vi "DeviceNet Display.vi"() -> ()   [LabVIEW 2011]
uses:
  Controls/DNet CommandRegister Cluster.ctl
  GlobalVariables.vi
panel:
  in  "Enable Write":bool
  out "DNET3":string
  out "DNET2":string
  out "DNET1":string
  in  "stop":bool
  in  "Reset":bool
  in  "HaltScanner":bool
  in  "DisableNetwork":bool
  in  "Fault":bool
  out "DnetPowerDetect":bool
  out "DupNodeFail":bool
  out "CommFailure":bool
  out "Autoverify":bool
  out "DeviceFailure":bool
  out "DisableNetwork":bool
  out "Fault":bool
  out "Run":bool
  in  "Run":bool
  in  "Reset":bool
  in  "HaltScanner":bool
  in  "DisableNetwork":bool
  in  "Fault":bool
  out "DnetPowerDetect":bool
  out "DupNodeFail":bool
  out "CommFailure":bool
  out "Autoverify":bool
  out "DeviceFailure":bool
  out "DisableNetwork":bool
  out "Fault":bool
  out "Run":bool
  in  "Run":bool
  in  "Reset":bool
  in  "HaltScanner":bool
  in  "DisableNetwork":bool
  in  "Fault":bool
  out "DnetPowerDetect":bool
  out "DupNodeFail":bool
  out "CommFailure":bool
  out "Autoverify":bool
  out "DeviceFailure":bool
  out "DisableNetwork":bool
  out "Fault":bool
  out "Run":bool
  in  "Run":bool
  # "DeviceNet 1"
  # "DeviceNet 2"
  # "DeviceNet 3"
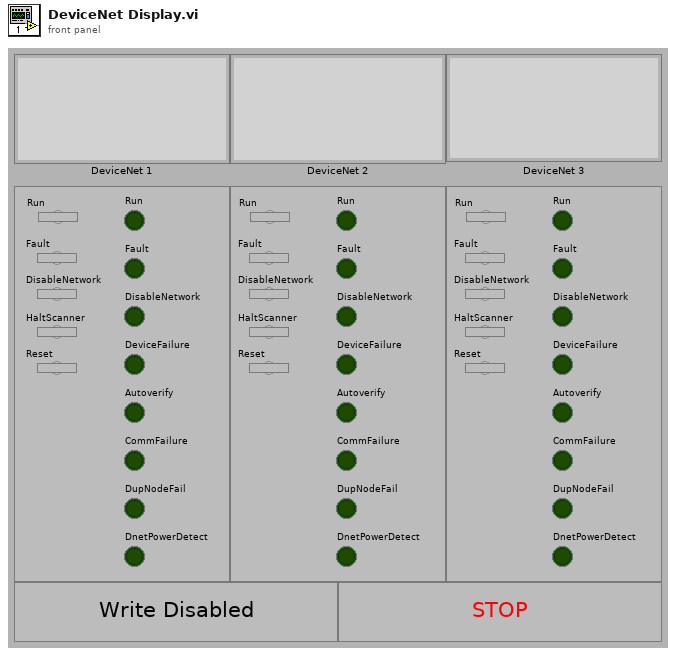
[diagram p1: front panel]
types:
  T1 = typedef "DNet CommandRegister Cluster.ctl" = cluster{"Run":bool, "Fault":bool, "DisableNetowrk":bool, "HaltScanner":bool, "Reset":bool}
  T2 = typedef "DNet StatusRegister Cluster.ctl" = cluster{"Run":bool, "Fault":bool, "DisableNetwork":bool, "DeviceFailure":bool, "Autoverify":bool, "CommFailure":bool, "DupNodeFail":bool, "DnetPowerDetect":bool}
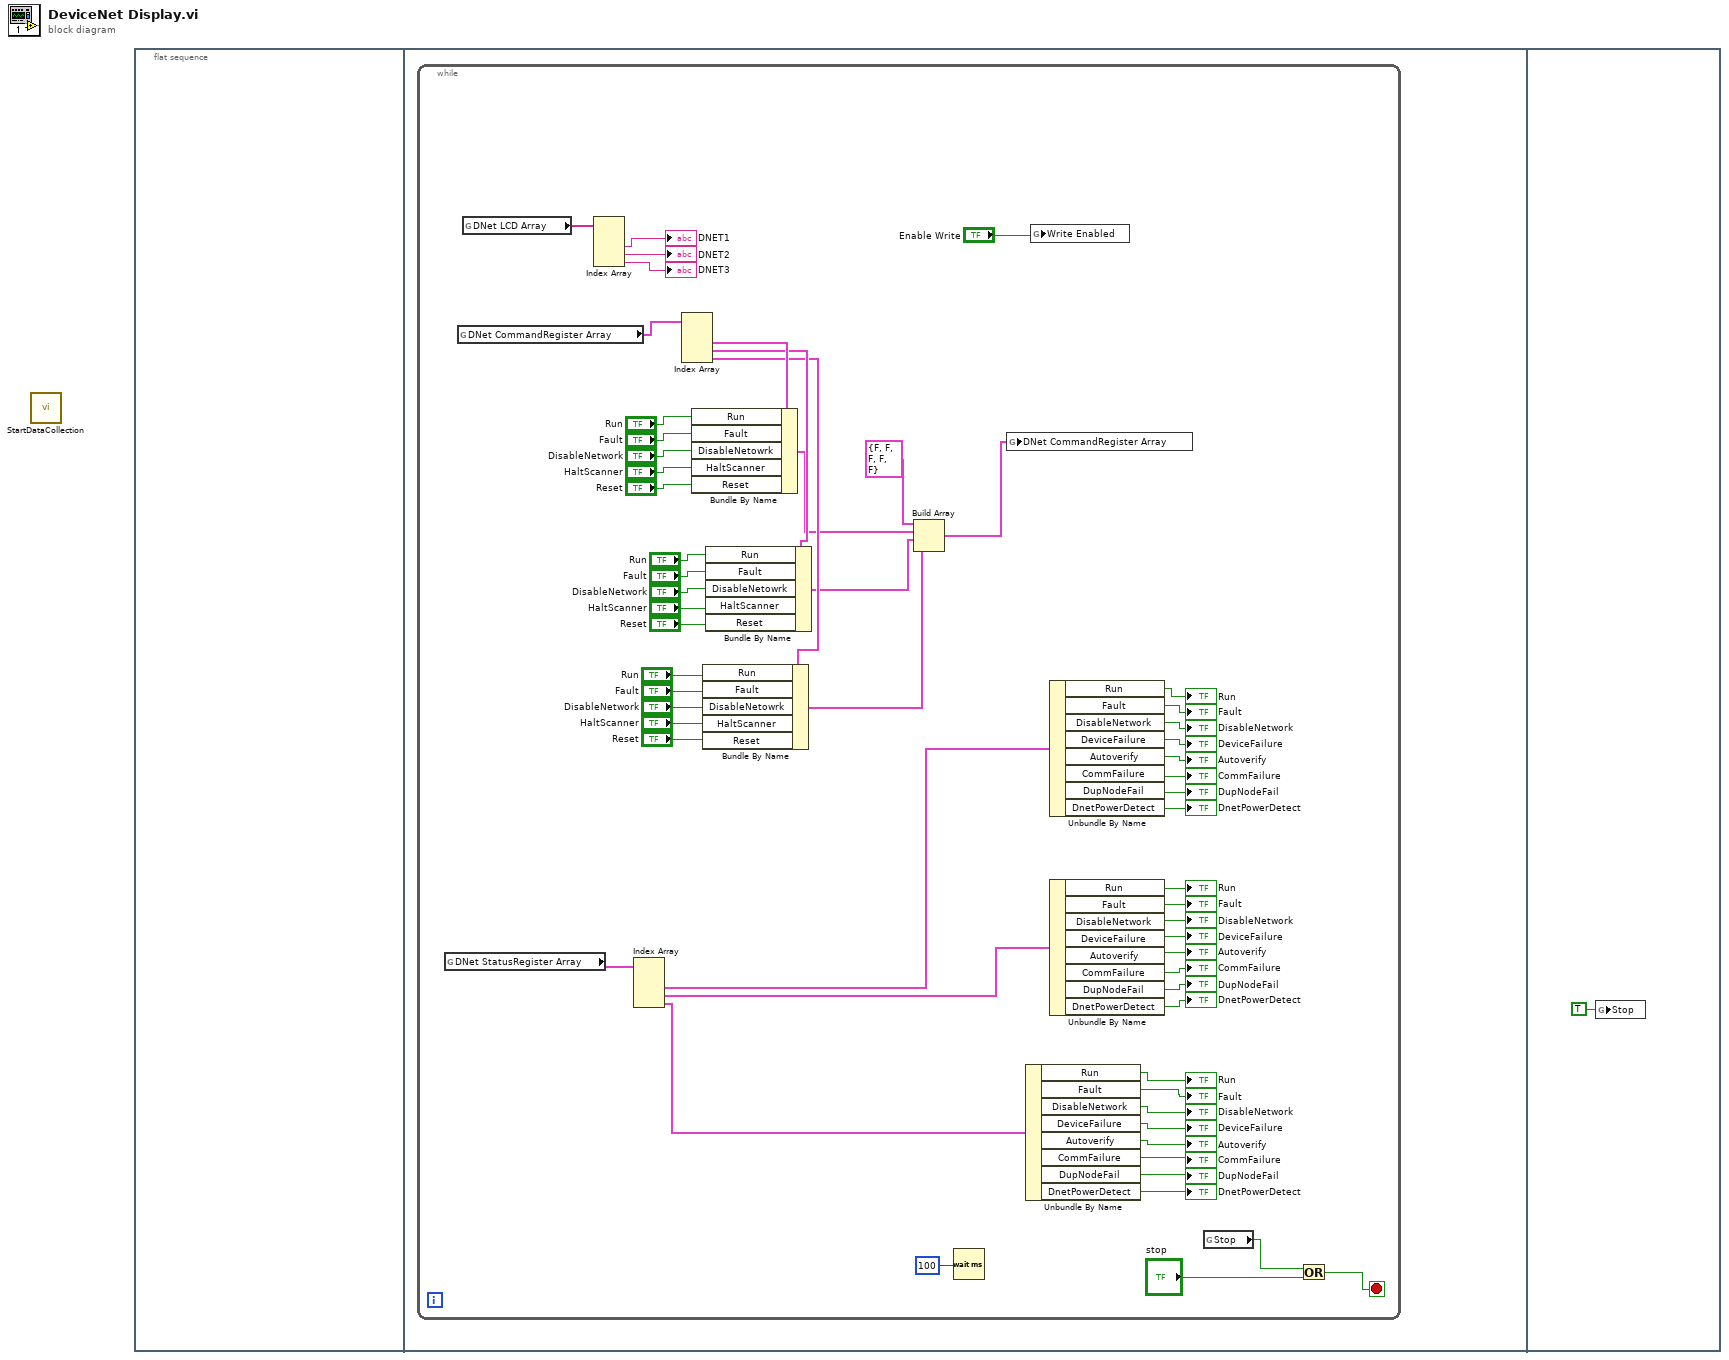
[diagram p0: block diagram]
diagram:
  n1 = call "StartDataCollection.vi"() -> ()  [unwired: 12 in]
  n2 = flat-sequence {
    frame #0 {
    }
    frame #1 {
      n3 = while {
        stop <- w2 stop-if-true
        n4 = global read "GlobalVariables.vi" "DNet StatusRegister Array"() -> (w33:T2[])
        n5 = global read "GlobalVariables.vi" "DNet CommandRegister Array"() -> (w55:T1[])
        n6 = global read "GlobalVariables.vi" "DNet LCD Array"() -> (w60:string[])
        n7 = Index Array(array=w60) -> (element #2=→"DNET1":string, element #3=→"DNET2":string, element #4=→"DNET3":string)  [unwired: 4 in, 1 out]
        n8 = Index Array(array=w33) -> (element #2=w32:T2, element #3=w31:T2, element #4=w30:T2)  [unwired: 4 in, 1 out]
        n9 = Index Array(array=w55) -> (element #2=w56:T1, element #3=w54:T1, element #4=w53:T1)  [unwired: 4 in, 1 out]
        n10 = Bundle By Name(cluster=w56, "Run"="Run", "Fault"="Fault", "DisableNetowrk"="DisableNetwork", "HaltScanner"="HaltScanner", "Reset"="Reset") -> (w37:T1)
        n11 = Bundle By Name(cluster=w53, "Run"="Run", "Fault"="Fault", "DisableNetowrk"="DisableNetwork", "HaltScanner"="HaltScanner", "Reset"="Reset") -> (w35:T1)
        n12 = Bundle By Name(cluster=w54, "Run"="Run", "Fault"="Fault", "DisableNetowrk"="DisableNetwork", "HaltScanner"="HaltScanner", "Reset"="Reset") -> (w36:T1)
        n13 = Build Array(T1 {"Run"=FALSE, "Fault"=FALSE, "DisableNetowrk"=FALSE, "HaltScanner"=FALSE, "Reset"=FALSE} ("element"), w37, w36, w35) -> (w34:T1[])
        n14 = Wait (ms)(milliseconds to wait=100) -> ()  [unwired: 1 out]
        n15 = global write "GlobalVariables.vi" "DNet CommandRegister Array"(w34) -> ()
        n16 = Unbundle By Name(w30) -> ("Run"=→"Run":bool, "Fault"=→"Fault":bool, "DisableNetwork"=→"DisableNetwork":bool, "DeviceFailure"=→"DeviceFailure":bool, "Autoverify"=→"Autoverify":bool, "CommFailure"=→"CommFailure":bool, "DupNodeFail"=→"DupNodeFail":bool, "DnetPowerDetect"=→"DnetPowerDetect":bool)
        n17 = global write "GlobalVariables.vi" "Write Enabled"("Enable Write") -> ()
        n18 = Unbundle By Name(w32) -> ("Run"=→"Run":bool, "Fault"=→"Fault":bool, "DisableNetwork"=→"DisableNetwork":bool, "DeviceFailure"=→"DeviceFailure":bool, "Autoverify"=→"Autoverify":bool, "CommFailure"=→"CommFailure":bool, "DupNodeFail"=→"DupNodeFail":bool, "DnetPowerDetect"=→"DnetPowerDetect":bool)
        n19 = Unbundle By Name(w31) -> ("Run"=→"Run":bool, "Fault"=→"Fault":bool, "DisableNetwork"=→"DisableNetwork":bool, "DeviceFailure"=→"DeviceFailure":bool, "Autoverify"=→"Autoverify":bool, "CommFailure"=→"CommFailure":bool, "DupNodeFail"=→"DupNodeFail":bool, "DnetPowerDetect"=→"DnetPowerDetect":bool)
        n20 = global read "GlobalVariables.vi" "Stop"() -> (w3:bool)
        n21 = Or(x=w3, y="stop") -> (x .or. y?=w2:bool)
      }
    }
    frame #2 {
      n22 = global write "GlobalVariables.vi" "Stop"(TRUE ("Stop")) -> ()
    }
  }
